vi "Core Prepare.vi"(8 "error in (no error)":errorcluster, 11 "CIFTemplateNode in":refnum<class "CIFCorePlugin.lvclass">) -> (0 "error out":errorcluster, 3 "CIFTemplateNode out":refnum<class "CIFCorePlugin.lvclass">, 5 "Transition to Run":bool)   [LabVIEW 2021, in "CIFCorePlugin.lvclass"]
uses:
  CIFCorePlugin.lvclass
  CIFCorePlugin.lvclass/CIFCorePlugin.ctl
  Typedef/Energized States.ctl
  CIFUtilities/CIFClocks/Time Management/System Time to External Time.vi
  Common/Utilities/Add Error.vi
  Common/Utilities/Append Error Location.vi
  Common/Typedef/Simple Error.ctl
  Common/CIFCoreCommon.lvlib
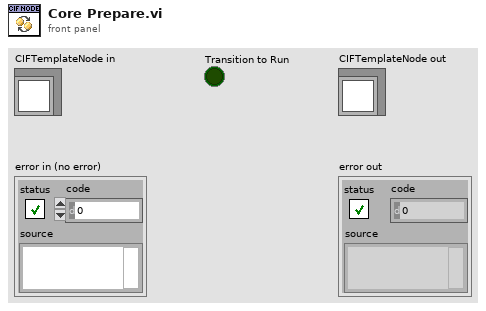
[diagram p1: front panel]
types:
  T1 = typedef "CIFCoreCommon.lvlib/Simple Error.ctl" = cluster{"status":bool, "code":i32}
  T2 = typedef "CIFCorePlugin.lvclass/Energized States.ctl" = enum16{"Listen", "Prepare", "Execute", "Housekeep", "Cleanup", "Destroy"}
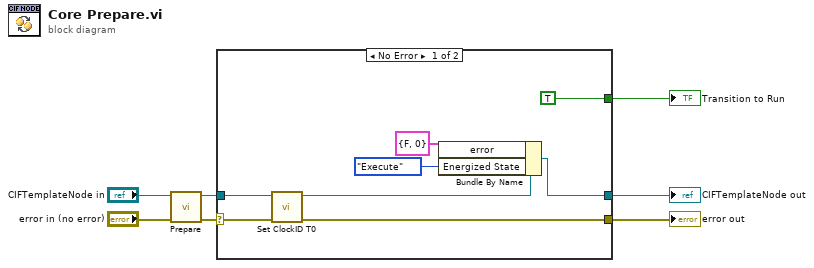
[diagram p0: block diagram]
diagram:
  n1 = call-dynamic "Prepare.vi"("error in (no error)"="error in (no error)", "CIFTemplateNode in"="CIFTemplateNode in") -> ("error out"=w3:errorcluster, "CIFTemplateNode out"=w1:refnum<class "CIFCorePlugin.lvclass">)  [unwired: 8 in]
  n2 = case shown="No Error" w3 {
    selector: w3 -> [w11 w17]
    tunnel: [w9 w17] -> w7
    tunnel: [w15 w16] -> w6
    tunnel: w1 -> [w12 w16]
    tunnel: [TRUE _] -> w5
    frame No Error {
      n3 = call "Set ClockID T0.vi"("error in (no error)"=w11, "CIFCorePlugin in"=w12) -> ("error out"=w9:errorcluster, "CIFCorePlugin out"=w10:refnum<class "CIFCorePlugin.lvclass">)  [unwired: 8 in]
      n4 = Bundle By Name(cluster=w10, "error"=T1 {"status"=FALSE, "code"=0} ("Status.error"), "Energized State"=Energized_States."Execute") -> (w15:refnum<class "CIFCorePlugin.lvclass">)
    }
    frame Error {
    }
  }
  "error out" <- w7
  "CIFTemplateNode out" <- w6
  "Transition to Run" <- w5
